vi "Write F4T .Net refnum.vi"(8 "error in (no error)":errorcluster, 10 "F4T .Net refnum":refnum<k24>, 11 "F4T in":refnum<class "F4T.lvclass">) -> (0 "error out":errorcluster, 3 "F4T out":refnum<class "F4T.lvclass">)   [LabVIEW 2018, in "F4T.lvlib" / "F4T.lvclass"]
uses:
  F4T.lvclass
  C:/Program Files/National Instruments/LabVIEW 2018/instr.lib/Watlow Std Bus/Public/Watbus.dll
  Program Files/National Instruments/LabVIEW 2018/instr.lib/Watlow Std Bus/Public/Watbus.dll
  F4T.lvclass/F4T.ctl
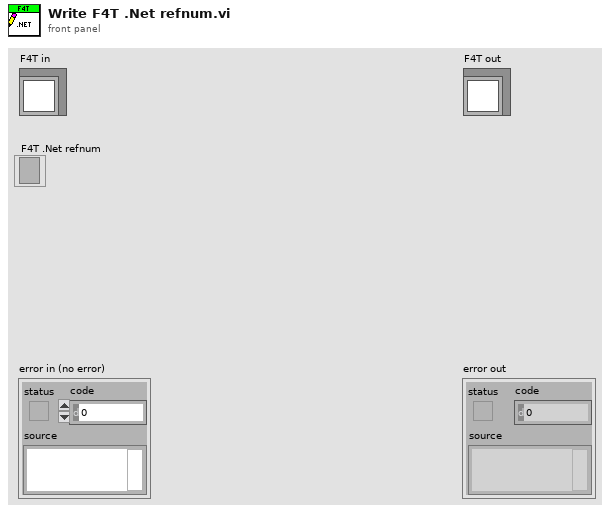
[diagram p1: front panel]
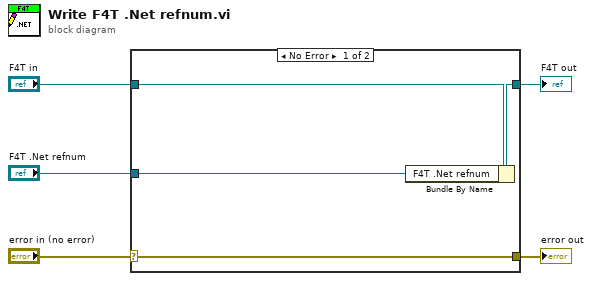
[diagram p0: block diagram]
diagram:
  n1 = case shown="No Error" "error in (no error)" {
    selector: "error in (no error)" -> [w9 w10]
    tunnel: [w9 w10] -> w4
    tunnel: [w7 w11] -> w2
    tunnel: "F4T in" -> [w8 w11]
    tunnel: "F4T .Net refnum" -> [w6 _]
    frame No Error {
      n2 = Bundle By Name(cluster=w8, "F4T .Net refnum"=w6) -> (w7:refnum<class "F4T.lvclass">)
    }
    frame Error {
    }
  }
  "error out" <- w4
  "F4T out" <- w2
